vi "Two_Try_Guessing_Game.vi"() -> ()   [LabVIEW 2022 SP3]
uses:
  <vilib>/numeric/Random Number (Range) I64.vi
  <vilib>/numeric/sub_Random U32.vi
panel:
  out "Message":string
  in  "OK Button":bool
  in  "User Guess":dbl
  # "Two Try Guessing Game:\nFollow the prompts to play this guessing game.\nYou will be given 2 chances to guess the right \nnumber from 1-10."
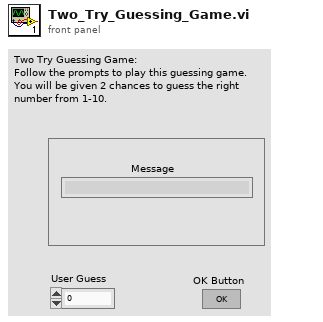
[diagram p1: front panel]
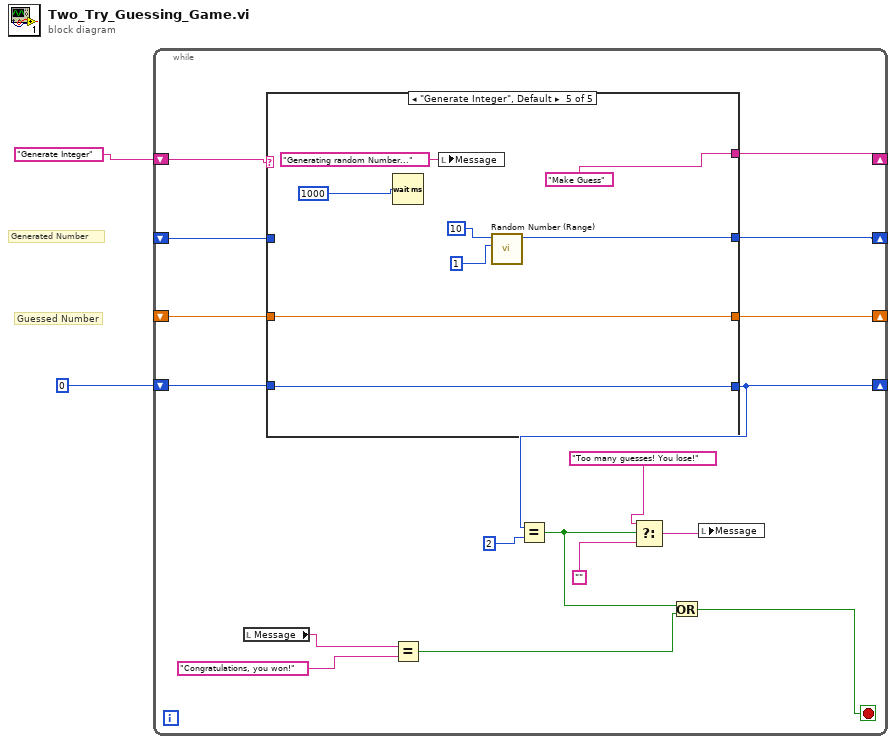
[diagram p0: block diagram]
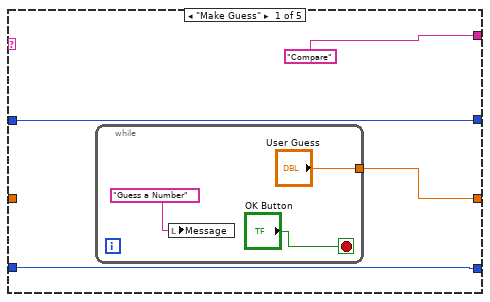
[diagram p2: hidden frame]
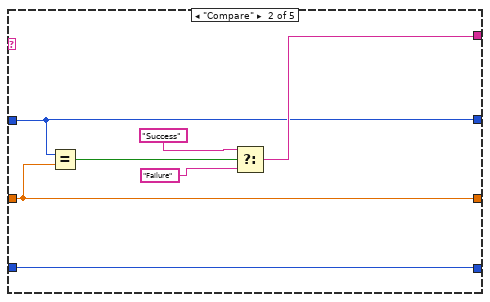
[diagram p3: hidden frame]
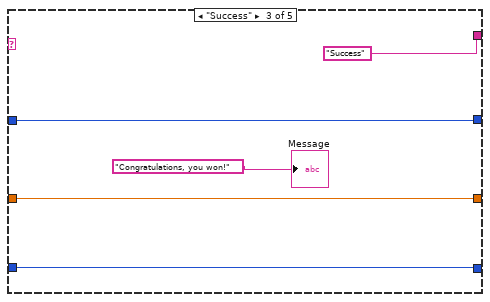
[diagram p4: hidden frame]
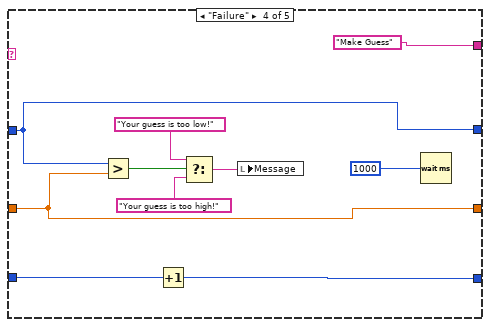
[diagram p5: hidden frame]
diagram:
  # "Guessed Number"
  # "Generated Number"
  n1 = while {
    shift-right: [w19] -> _
    shift-left: _ -> [w18]
    shift-right: [w17] -> _
    shift-left: _ -> [w16]
    shift-right: [w15] -> _
    shift-left: "Generate Integer" -> [w14]
    shift-right: [w3] -> _
    shift-left: 0 -> [w13]
    stop <- w9 stop-if-true
    n2 = local read "Message"() -> (w11:string)
    n3 = case shown="\"Generate Integer\", Default" w14 {
      tunnel: [w23 w29 w34 w42 w51] -> w19
      tunnel: w18 -> [w23 w29 w34 w42 _]
      tunnel: [w22 w28 w35 w43 w52] -> w17
      tunnel: w16 -> [_ w28 w35 w43 w52]
      tunnel: ["Compare" w30 "Success" "Make Guess" "Make Guess"] -> w15
      tunnel: w13 -> [w20 w27 w36 w44 w53]
      tunnel: [w20 w27 w36 w40 w53] -> w3
      frame "Make Guess" {
        n4 = while {
          tunnel: ["User Guess"] -> w22
          stop <- "OK Button" stop-if-true
          n5 = local write "Message"("Guess a Number") -> ()
        }
      }
      frame "Compare" {
        n6 = Equal?(x=w29, y=w28) -> (x = y?=w33:bool)
        n7 = Select(t="Success", s=w33, f="Failure") -> (s? t:f=w30:string)
      }
      frame "Success" {
        "Message" <- "Congratulations, you won!"
      }
      frame "Failure" {
        n8 = Greater?(x=w42, y=w43) -> (0:w48:bool)
        n9 = Increment(x=w44) -> (x+1=w40:i32)
        n10 = Select(t="Your guess is too low!", s=w48, f="Your guess is too high!") -> (s? t:f=w45:string)
        n11 = local write "Message"(w45) -> ()
        n12 = Wait (ms)(milliseconds to wait=1000) -> ()  [unwired: 1 out]
      }
      frame "Generate Integer", Default {
        n13 = Wait (ms)(milliseconds to wait=1000) -> ()  [unwired: 1 out]
        n14 = local write "Message"("Generating random Number...") -> ()
        n15 = call-poly <vilib>:"Random Number (Range).vi"("lower bound (-100)"=1, "upper bound (100)"=10) -> ("number"=w51:i64)  [unwired: 9 in]
      }
    }
    n16 = Equal?(x=w11, y="Congratulations, you won!") -> (x = y?=w12:bool)
    n17 = Equal?(x=w3, y=2) -> (x = y?=w7:bool)
    n18 = Select(t="Too many guesses! You lose!", s=w7, f="") -> (s? t:f=w5:string)
    n19 = Or(x=w7, y=w12) -> (x .or. y?=w9:bool)
    n20 = local write "Message"(w5) -> ()
  }
